vi "DSF Config File to Engine Config Cluster.vi"(8 "error in (no error)":errorcluster, 11 "dsf configuration file path":path) -> (0 "error out":errorcluster, 3 "framework configuration out":T1)   [LabVIEW 2017, in "DSF Core.lvlib" / "Configuration Session.lvclass"]
uses:
  Configuration/Configuration Session.lvclass
  Configuration/Public/Controls/DSF Engine Framework Configuration.ctl
  Configuration/Public/Controls/DSF Engine Plugin Configuration.ctl
  Configuration/Public/Controls/DSF Timing Info.ctl
  Configuration/Public/Controls/DSF Engine Transfer Group Configuration.ctl
  Configuration/Public/Controls/DSF Direction.ctl
  Configuration/Public/Controls/DSF Engine Transfer Configuration.ctl
  Configuration/Public/Controls/DSF Byte Order.ctl
  Configuration/Public/Controls/DSF Engine Channel Configuration.ctl
  Configuration/Public/Controls/DSF Data Type.ctl
  Configuration/Public/Controls/DSF Settings Info.ctl
  Configuration/Public/Read All Item IDs/Read All Plugin IDs.vi
  Configuration/Public/Read Item/Read Plugin.vi
  Configuration/Public/Read Item/Read Settings.vi
  Configuration/Public/Read Item/Read Group.vi
  Configuration/Public/Read Item/Read Transfer.vi
  Configuration/Public/Read Item/Read Channel.vi
  DSF Core.lvlib
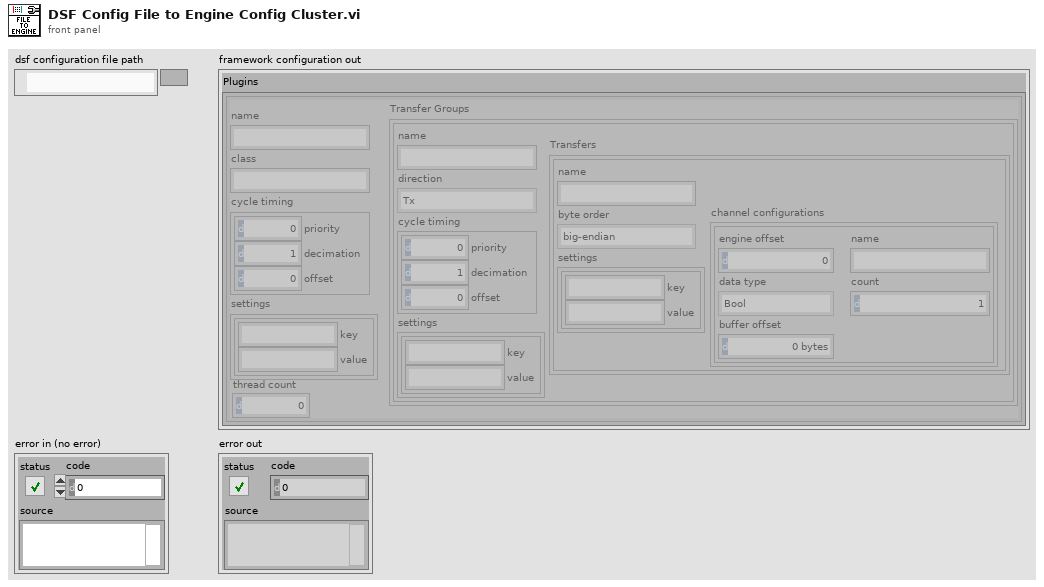
[diagram p1: front panel]
types:
  T1 = typedef "DSF Core.lvlib/DSF Engine Framework Configuration.ctl" = cluster{"Plugins":T2[]}
  T2 = typedef "DSF Core.lvlib/DSF Engine Plugin Configuration.ctl" = cluster{"name":string, "class":string, "cycle timing":T3, "Transfer Groups":T4[], "settings":T10, "thread count":i32}
  T3 = typedef "DSF Core.lvlib/DSF Timing Info.ctl" = cluster{"priority":u64, "decimation":u64, "offset":u64}
  T4 = typedef "DSF Core.lvlib/DSF Engine Transfer Group Configuration.ctl" = cluster{"name":string, "direction":T5, "cycle timing":T3, "Transfers":T6[], "settings":T10}
  T5 = typedef "DSF Core.lvlib/DSF Direction.ctl" = enum8{"Tx", "Rx"}
  T6 = typedef "DSF Core.lvlib/DSF Engine Transfer Configuration.ctl" = cluster{"name":string, "byte order":T7, "channel configurations":T8[], "settings":T10}
  T7 = typedef "DSF Core.lvlib/DSF Byte Order.ctl" = enum8{"big-endian", "little-endian"}
  T8 = typedef "DSF Core.lvlib/DSF Engine Channel Configuration.ctl" = cluster{"engine offset":u64, "name":string, "data type":T9, "count":u64, "buffer offset":u64}
  T9 = typedef "DSF Core.lvlib/DSF Data Type.ctl" = enum8{"Bool", "SGL", "DBL", "I8", "I16", "I32", "I64", "U8", "U16", "U32", "U64"}
  T10 = typedef "DSF Core.lvlib/DSF Settings Info.ctl" = cluster{"key":string, "value":string}[]
  T11 = typedef "DSF Core.lvlib/DSF Plugin Info.ctl" = cluster{"type":string, "timing":T3, "group ids":string[], "settings id":string, "thread count":i32}
  T12 = typedef "DSF Core.lvlib/DSF Group Info.ctl" = cluster{"direction":T5, "timing":T3, "transfer ids":string[], "settings id":string}
  T13 = typedef "DSF Core.lvlib/DSF Transfer Info.ctl" = cluster{"byte order":T7, "channel ids":string[], "settings id":string}
  T14 = typedef "DSF Core.lvlib/DSF Channel Info.ctl" = cluster{"count":u64, "buffer offset":u64, "data type":T9, "settings id":string}
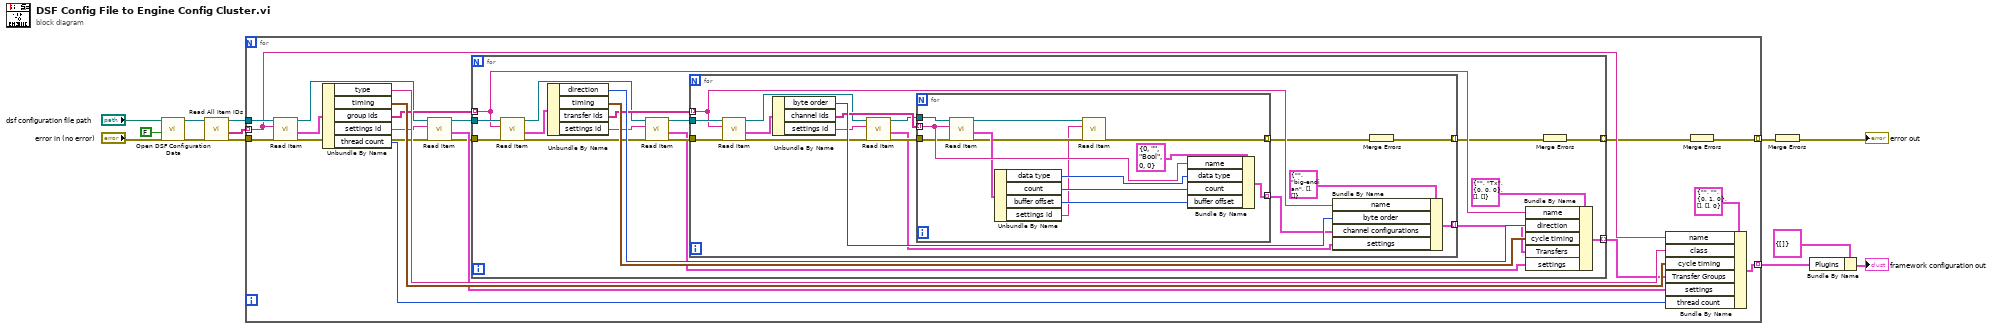
[diagram p0: block diagram]
diagram:
  n1 = call "Open DSF Configuration Data.vi"("error in (no error)"="error in (no error)", "replace if found? (F)"=FALSE ("create file if necessary (T)"), "dsf configuration file path"="dsf configuration file path") -> ("error out"=w4:errorcluster, "Configuration Session"=w5:refnum<class "Configuration Session.lvclass">)  [unwired: 4 in, 3 out]
  n2 = call-poly "Read All Item IDs.vi"("error in (no error)"=w4, "Configuration Session in"=w5) -> ("error out"=w10:errorcluster, "Plugin IDs"=w12:string[], "Configuration Session out"=w11:refnum<class "Configuration Session.lvclass">)  [unwired: 7 in]
  n3 = for {
    tunnel: w12 -> [w24] mode=indexing
    tunnel: w11 -> [w31]
    tunnel: [w27] -> w6 mode=indexing
    tunnel: w10 -> [w18]
    tunnel: [w15] -> w9 mode=indexing
    n4 = call-poly "Read Item.vi"("error in (no error)"=w18, "Plugin ID"=w24, "Configuration Session in"=w31) -> ("error out"=w19:errorcluster, "value"=w30:T11, "Configuration Session out"=w23:refnum<class "Configuration Session.lvclass">)  [unwired: 5 in, 1 out]
    n5 = Unbundle By Name(w30) -> ("type"=w29:string, "timing"=w28:T3, "group ids"=w26:string[], "settings id"=w21:string, "thread count"=w14:i32)
    n6 = call-poly "Read Item.vi"("error in (no error)"=w19, "Settings ID"=w21, "Configuration Session in"=w23) -> ("error out"=w17:errorcluster, "value"=w20:T10, "Configuration Session out"=w22:refnum<class "Configuration Session.lvclass">)  [unwired: 5 in, 1 out]
    n7 = for {
      tunnel: w22 -> [w50]
      tunnel: w26 -> [w47] mode=indexing
      tunnel: [w44] -> w25 mode=indexing
      tunnel: w17 -> [w41]
      tunnel: [w33] -> w16 mode=indexing
      n8 = call-poly "Read Item.vi"("error in (no error)"=w41, "Group ID"=w47, "Configuration Session in"=w50) -> ("error out"=w37:errorcluster, "value"=w48:T12, "Configuration Session out"=w40:refnum<class "Configuration Session.lvclass">)  [unwired: 5 in, 1 out]
      n9 = Unbundle By Name(w48) -> ("direction"=w46:T5, "timing"=w45:T3, "transfer ids"=w43:string[], "settings id"=w38:string)
      n10 = call-poly "Read Item.vi"("error in (no error)"=w37, "Settings ID"=w38, "Configuration Session in"=w40) -> ("error out"=w36:errorcluster, "value"=w35:T10, "Configuration Session out"=w39:refnum<class "Configuration Session.lvclass">)  [unwired: 5 in, 1 out]
      n11 = for {
        tunnel: w43 -> [w60] mode=indexing
        tunnel: w39 -> [w67]
        tunnel: [w64] -> w42 mode=indexing
        tunnel: w36 -> [w59]
        tunnel: [w52] -> w34 mode=indexing
        n12 = call-poly "Read Item.vi"("error in (no error)"=w59, "Transfer ID"=w60, "Configuration Session in"=w67) -> ("error out"=w57:errorcluster, "value"=w66:T13, "Configuration Session out"=w61:refnum<class "Configuration Session.lvclass">)  [unwired: 5 in, 1 out]
        n13 = Unbundle By Name(w66) -> ("byte order"=w65:T7, "channel ids"=w62:string[], "settings id"=w56:string)
        n14 = call-poly "Read Item.vi"("error in (no error)"=w57, "Settings ID"=w56, "Configuration Session in"=w61) -> ("error out"=w55:errorcluster, "value"=w54:T10, "Configuration Session out"=w58:refnum<class "Configuration Session.lvclass">)  [unwired: 5 in, 1 out]
        n15 = for {
          tunnel: [w80] -> w63 mode=indexing
          tunnel: w62 -> [w78] mode=indexing
          tunnel: w58 -> [w79]
          tunnel: w55 -> [w73]
          tunnel: [w69] -> w53 mode=indexing
          n16 = call-poly "Read Item.vi"("error in (no error)"=w73, "Channel ID"=w78, "Configuration Session in"=w79) -> ("error out"=w71:errorcluster, "value"=w77:T14, "Configuration Session out"=w72:refnum<class "Configuration Session.lvclass">)  [unwired: 5 in, 1 out]
          n17 = Unbundle By Name(w77) -> ("data type"=w76:T9, "count"=w75:u64, "buffer offset"=w74:u64, "settings id"=w70:string)
          n18 = call-poly "Read Item.vi"("error in (no error)"=w71, "Settings ID"=w70, "Configuration Session in"=w72) -> ("error out"=w69:errorcluster)  [unwired: 5 in, 3 out]
          n19 = Bundle By Name(cluster=T8 {"engine offset"=0, "name"="", "data type"=enum."Bool", "count"=0, "buffer offset"=0} ("channel configurations"), "name"=w78, "data type"=w76, "count"=w75, "buffer offset"=w74) -> (w80:T8)
        }
        n20 = Bundle By Name(cluster=T6 {"name"="", "byte order"=enum."big-endian", "channel configurations"=[], "settings"=[]} ("Transfer Configuration"), "name"=w60, "byte order"=w65, "channel configurations"=w63, "settings"=w54) -> (w64:T6)
        n21 = Merge Errors(w53) -> (w52:errorcluster)
      }
      n22 = Bundle By Name(cluster=T4 {"name"="", "direction"=enum."Tx", "cycle timing"={"priority"=0, "decimation"=0, "offset"=0}, "Transfers"=[], "settings"=[]} ("Transfer Group Configuration"), "name"=w47, "direction"=w46, "cycle timing"=w45, "Transfers"=w42, "settings"=w35) -> (w44:T4)
      n23 = Merge Errors(w34) -> (w33:errorcluster)
    }
    n24 = Bundle By Name(cluster=T2 {"name"="", "class"="", "cycle timing"={"priority"=0, "decimation"=1, "offset"=0}, "Transfer Groups"=[], "settings"=[], "thread count"=0} ("Plugin Configuration"), "name"=w24, "class"=w29, "cycle timing"=w28, "Transfer Groups"=w25, "settings"=w20, "thread count"=w14) -> (w27:T2)
    n25 = Merge Errors(w16) -> (w15:errorcluster)
  }
  n26 = Merge Errors(w9) -> (→"error out":errorcluster)
  n27 = Bundle By Name(cluster=T1 {"Plugins"=[]} ("Framework Config (JSON)"), "Plugins"=w6) -> (→"framework configuration out":T1)
